vi "Offset Channel Index.vi"() -> (0 "index":i32)   [LabVIEW 2021]
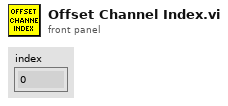
[diagram p1: front panel]
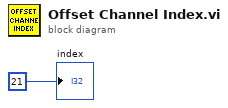
[diagram p0: block diagram]
diagram:
  "index" <- 21 ("index")
